vi "Write Frequency.vi"(8 "error in (no error)":errorcluster, 10 "Frequency":dbl, 11 "Protocols in":refnum<class "Protocols.lvclass">) -> (0 "error out":errorcluster, 3 "Protocols out":refnum<class "Protocols.lvclass">)   [LabVIEW 2020, in "I2C Controller.lvlib" / "Protocols.lvclass"]
uses:
  Protocols.lvclass
  Protocols.lvclass/Protocols.ctl
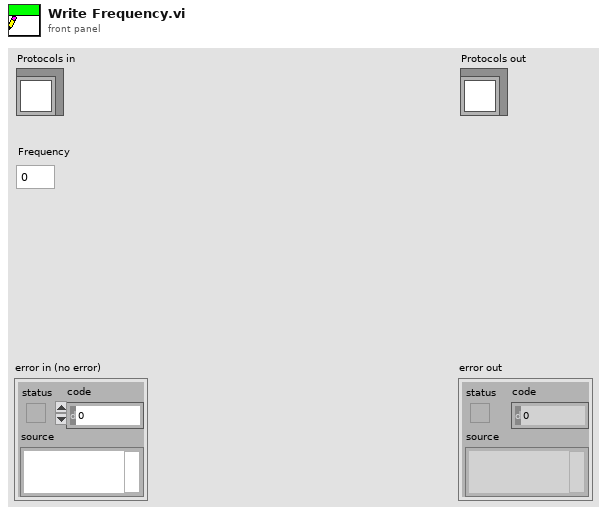
[diagram p1: front panel]
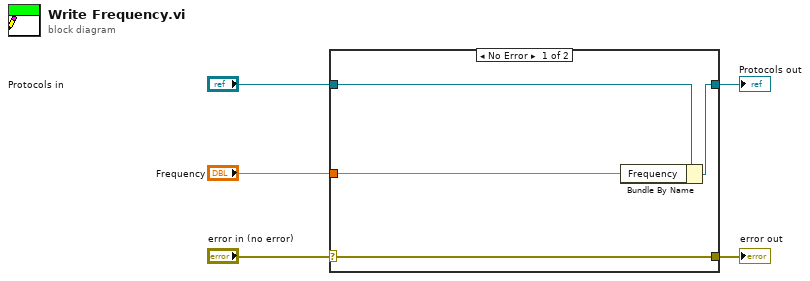
[diagram p0: block diagram]
diagram:
  n1 = case shown="No Error" "error in (no error)" {
    selector: "error in (no error)" -> [w9 w10]
    tunnel: [w9 w10] -> w4
    tunnel: [w7 w11] -> w2
    tunnel: "Protocols in" -> [w8 w11]
    tunnel: "Frequency" -> [w6 _]
    frame No Error {
      n2 = Bundle By Name(cluster=w8, "Frequency"=w6) -> (w7:refnum<class "Protocols.lvclass">)
    }
    frame Error {
    }
  }
  "error out" <- w4
  "Protocols out" <- w2
